vi "Generate container from FQN.vi"(8 "error in (no error)":errorcluster, 11 "Fully Qualified Name":string) -> (0 "error out":errorcluster, 2 "Unowned?":bool, 3 "DGML Strings":string[](array[string]))   [LabVIEW 2018, in "DGML creation.lvlib"]
uses:
  DGML creation.lvlib
  Path and string processing/Path and String Processing.lvlib
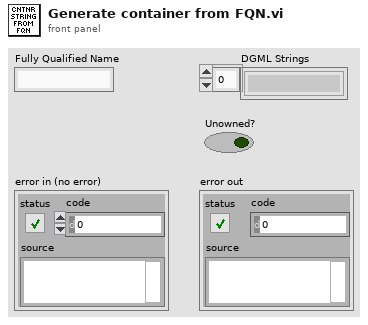
[diagram p1: front panel]
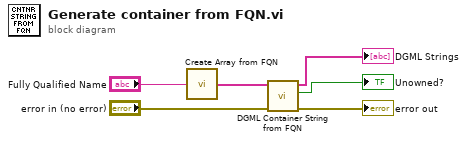
[diagram p0: block diagram]
diagram:
  n1 = call "Create Array from FQN.vi"("FQN In"="Fully Qualified Name") -> ("Array of namespaces and name"=w1:string[])
  n2 = call "DGML Container String from FQN.vi"("error in (no error)"="error in (no error)", "FQN Array"=w1) -> ("error out"=→"error out":errorcluster, "Unowned?"=→"Unowned?":bool, "DGML Strings"=→"DGML Strings":string[])  [unwired: 7 in]
